vi "Get Values.vi"(8 "error in (no error)":errorcluster, 11 "Section in":refnum<class "Section.lvclass">) -> (0 "error out":errorcluster, 2 "Values":refnum<class "Value.lvclass">[](array[class]), 3 "Section out":refnum<class "Section.lvclass">)   [LabVIEW 2019, in "Electronic Datasheet.lvlib" / "Section.lvclass"]
uses:
  Section.lvclass
  Value/Value.lvclass
  Section.lvclass/Section.ctl
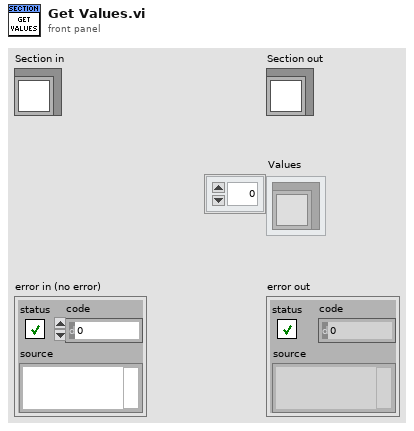
[diagram p1: front panel]
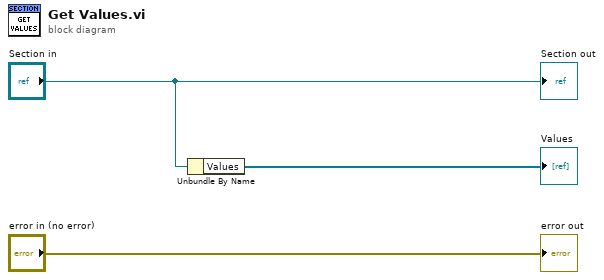
[diagram p0: block diagram]
diagram:
  n1 = Unbundle By Name("Section in") -> ("Values"=→"Values":refnum<class "Value.lvclass">[])
  "error out" <- "error in (no error)"
  "Section out" <- "Section in"
